vi "CPP-BLCompareToTarget.vi"() -> (0 "New Values In":string[][](array[string]), 1 "New Chs In":string[](array[string]))   [LabVIEW 2018]
uses:
  Results_plotter_Global.vi
  Data plotting/subVIs/Plot_Values_Global.vi
panel:
  out "Channel names":string[](array[string])
  in  "TargetSource":enum16{"First Profile", "Front Panel"}(ring)
  in  "aTarget":cluster{"Xvalues":dbl[], "Yvalues":dbl[]}={"Xvalues"=[1.040926042556437, 1.0312252179740482, 1.0211896176877788, 1.0107916504073806, 1.0, 0.9887789066622864, 0.9770872631810879, 0.9648774654735645, 0.9520939317160783, 0.9386711670518244, 0.9245311936078002, 0.9095800754352008, 0.8937031220268912, 0.8767581097958107, 0.8585654364377537, 0.8388933525508411, 0.8174349420135516, 0.7937705277401984, 0.7673026110088009, 0.7371346086455506], "Yvalues"=[600.0, 575.0, 550.0, 525.0, 500.0, 475.0, 450.0, 425.0, 400.0, 375.0, 350.0, 325.0, 300.0, 275.0, 250.0, 225.0, 200.0, 175.0, 150.0, 125.0]}
  in  "Zref":dbl=450.0
  # "This VI receives \"classic\" transposed plots of U (raw or normlised) vs Z, and linearly interpolates to find a velocites at the heights of the target data. It then computes error between the measured and target profiles.\nAlso works for TI, when normalisation will automatically be turned off"
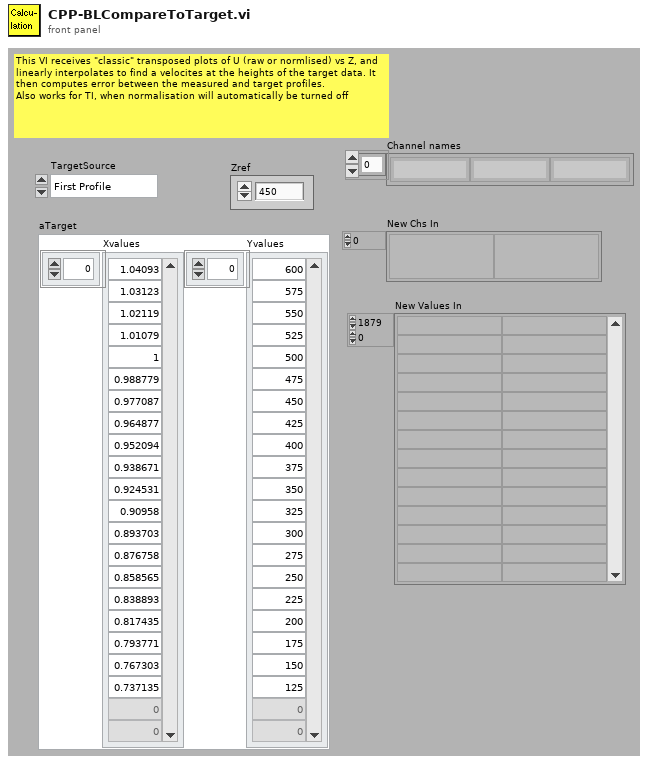
[diagram p1: front panel]
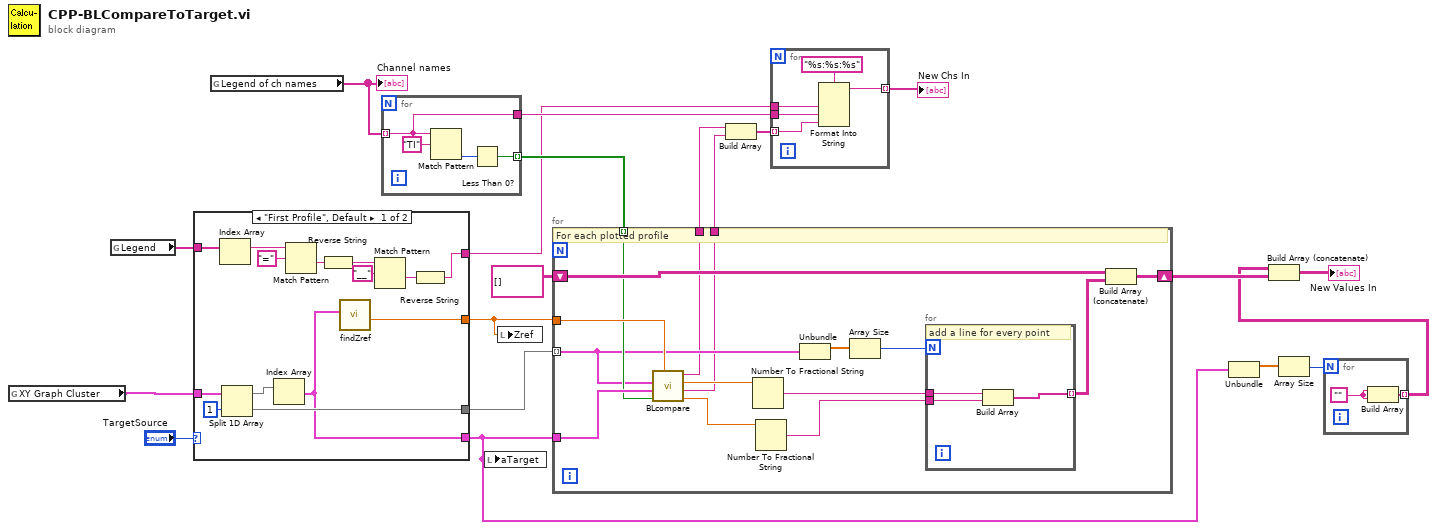
[diagram p0: block diagram]
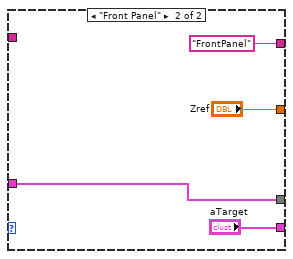
[diagram p2: hidden frame]
diagram:
  n1 = global read "Plot_Values_Global.vi" "XY Graph Cluster"() -> (w1:cluster{dbl[], dbl[]}[])
  n2 = global read "Results_plotter_Global.vi" "Legend"() -> (w11:string[])
  n3 = case shown="\"First Profile\", Default" "TargetSource" {
    tunnel: [w30 "aTarget"] -> w6
    tunnel: w1 -> [w34 w37]
    tunnel: [w31 w37] -> w17
    tunnel: [w29 "Zref"] -> w16
    tunnel: [w21 "FrontPanel"] -> w10
    tunnel: w11 -> [w23 _]
    frame "First Profile", Default {
      n4 = Index Array(array=w23) -> (element=w22:string)  [unwired: 1 in]
      n5 = Split 1D Array(array=w34, index=1) -> (first subarray=w33:cluster{dbl[], dbl[]}[], second subarray=w31:cluster{dbl[], dbl[]}[])
      n6 = Index Array(array=w33) -> (element=w30:cluster{dbl[], dbl[]})  [unwired: 1 in]
      n7 = Match Pattern(string=w22, regular expression="=") -> (after substring=w27:string)  [unwired: 1 in, 3 out]
      n8 = Reverse String(1:w27) -> (0:w25:string)
      n9 = call "findZref.vi"("aTarget"=w30) -> ("Zref"=w29:dbl)  [unwired: 10 in]
      n10 = Match Pattern(string=w25, regular expression="__") -> (after substring=w24:string)  [unwired: 1 in, 3 out]
      n11 = Reverse String(1:w24) -> (0:w21:string)
    }
    frame "Front Panel" {
    }
  }
  n12 = global read "Results_plotter_Global.vi" "Legend of ch names"() -> (w15:string[])
  "Channel names" <- w15
  n13 = for {
    tunnel: w15 -> [w39] mode=indexing
    tunnel: [w40] -> w14 mode=indexing
    tunnel: [w39] -> w13
    n14 = Match Pattern(string=w39, regular expression="TI") -> (offset past match=w41:i32)  [unwired: 1 in, 3 out]
    n15 = Less Than 0?(x=w41) -> (x < 0?=w40:bool)
  }
  n16 = local write "aTarget"(w6) -> ()
  n17 = local write "Zref"(w16) -> ()
  n18 = for {
    tunnel: w16 -> [w51]
    tunnel: w17 -> [w46] mode=indexing
    shift-right: [w56] -> w19
    shift-left: string[][] [] -> [w55]
    tunnel: w6 -> [w48]
    tunnel: w14 -> [w47] mode=indexing
    tunnel: [w44] -> w4
    tunnel: [w43] -> w3
    # "For each plotted profile"
    n19 = call "BLcompare.vi"("Zref"=w51, "Normalise?"=w47, "aTarget"=w48, "aSeries"=w46) -> ("metric2value"=w45:dbl, "metric2name"=w43:string, "metric1value"=w50:dbl, "metric1name"=w44:string)  [unwired: 4 in]
    n20 = Number To Fractional String(number=w50) -> (F-format string=w57:string)  [unwired: 3 in]
    n21 = Number To Fractional String(number=w45) -> (F-format string=w49:string)  [unwired: 3 in]
    n22 = Unbundle(w46) -> (w53:dbl[])  [unwired: 1 out]
    n23 = Array Size(array=w53) -> (size(s)=w54:i32)
    n24 = for {
      N: w54 -> [_]
      tunnel: w57 -> [w60]
      tunnel: [w59] -> w52 mode=indexing
      tunnel: w49 -> [w58]
      # "add a line for every point"
      n25 = Build Array(w60, w58) -> (w59:string[])
    }
    n26 = Build Array (concatenate)(w55, w52) -> (w56:string[][])
  }
  n27 = Build Array(w4, w3) -> (w2:string[])
  n28 = for {
    tunnel: w13 -> [w64]
    tunnel: [w65] -> w12 mode=indexing
    tunnel: w10 -> [w63]
    tunnel: w2 -> [w62] mode=indexing
    n29 = Format Into String(format string="%s:%s:%s", w63, w64, w62) -> (resulting string=w65:string)  [unwired: 2 in, 1 out]
  }
  "New Chs In" <- w12
  n30 = Unbundle(w6) -> ("Xvalues"=w8:dbl[])  [unwired: 1 out]
  n31 = Array Size(array=w8) -> (size(s)=w7:i32)
  n32 = for {
    N: w7 -> [_]
    tunnel: [w66] -> w5 mode=indexing
    w67 = "" ("element")
    n33 = Build Array(w67, w67) -> (w66:string[])
  }
  n34 = Build Array (concatenate)(w5, w19) -> (→"New Values In":string[][])
